vi "Write Task Into Map.vi"(8 "error in (no error)":errorcluster, 9 "Task In":refnum<class "Task Ancestor.lvclass">, 10 "Key":i64, 11 "Composite Map Task in":refnum<class "Composite Map Task.lvclass">) -> (0 "error out":errorcluster, 3 "Composite Map Task out":refnum<class "Composite Map Task.lvclass">)   [LabVIEW 2022 SP3, in "Composite Map Task.lvclass"]
uses:
  Composite Map Task.lvclass
  Task Ancestor/Task Ancestor.lvclass
  Composite Map Task.lvclass/Composite Map Task.ctl
  <vilib>/Utility/miscctls.llb/LVMapReplaceAction.ctl
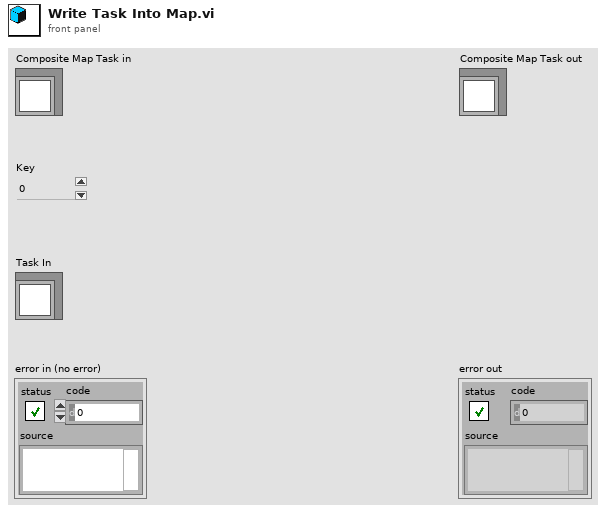
[diagram p1: front panel]
types:
  T1 = typedef "LVMapReplaceAction.ctl" = enum32{"Modify Entry only if found", "Add or Modify Entry", "Delete Entry"}
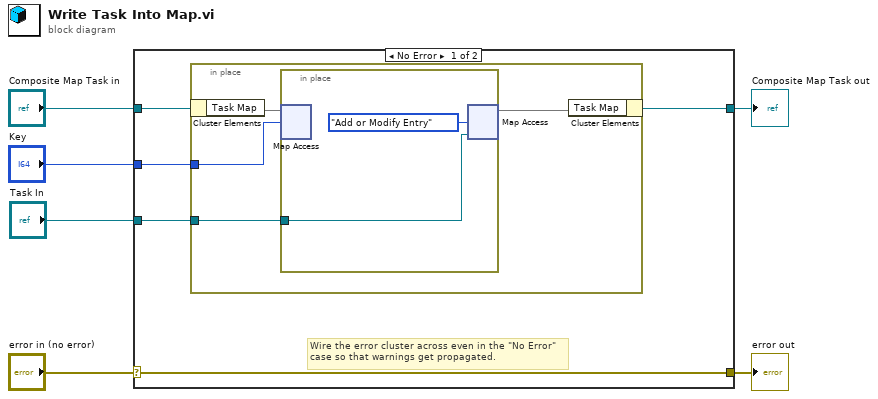
[diagram p0: block diagram]
diagram:
  n1 = case shown="No Error" "error in (no error)" {
    selector: "error in (no error)" -> [w11 w19]
    tunnel: [w11 w19] -> w5
    tunnel: [w9 w18] -> w3
    tunnel: "Composite Map Task in" -> [w10 w18]
    tunnel: "Key" -> [w8 _]
    tunnel: "Task In" -> [w7 _]
    frame No Error {
      # "Wire the error cluster across even in the \"No Error\"\ncase so that warnings get propagated."
      n2 = in-place {
        in-place-border: w8 -> [w13]
        in-place-border: w7 -> [w12]
        n3 = in-place-cluster #1(w10) -> ("Task Map"=w15:map{i64, refnum<class "Task Ancestor.lvclass">})
        n4 = in-place {
          in-place-border: w12 -> [w16]
          n5 = in-place-map #2(w15, w13) -> ()  [unwired: 1 in, 2 out]
          n6 = in-place-map #2(w16, LVMapReplaceAction."Add or Modify Entry" ("action")) -> (w14:map{i64, refnum<class "Task Ancestor.lvclass">})  [unwired: 2 out]
        }
        n7 = in-place-cluster #1("Task Map"=w14) -> (w9:refnum<class "Composite Map Task.lvclass">)
      }
    }
    frame Error {
    }
  }
  "error out" <- w5
  "Composite Map Task out" <- w3
